vi "Receive Control Drop Event.vi"(8 "error in (no error)":errorcluster, 10 "ControlDropMsg":refnum<class "ControlDropMsg.lvclass">, 11 "IEventAggregator In":refnum<class "IEventAggregator.lvclass">) -> (0 "error out":errorcluster, 3 "IEventAggregator Out":refnum<class "IEventAggregator.lvclass">)   [LabVIEW 2020, in "ActorEvents.lvlib" / "IEventAggregator.lvclass"]
doc: "抽象方法\n接收控件放置事件"
uses:
  IEventAggregator.lvclass
  IEventAggregator Messages/ControlDropMsg/ControlDropMsg.lvclass
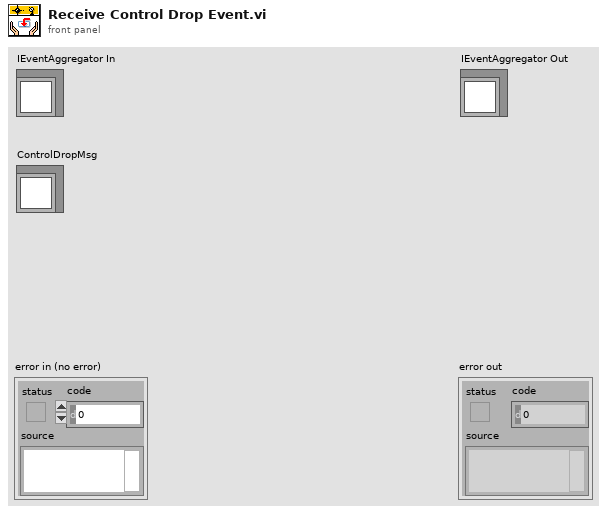
[diagram p1: front panel]
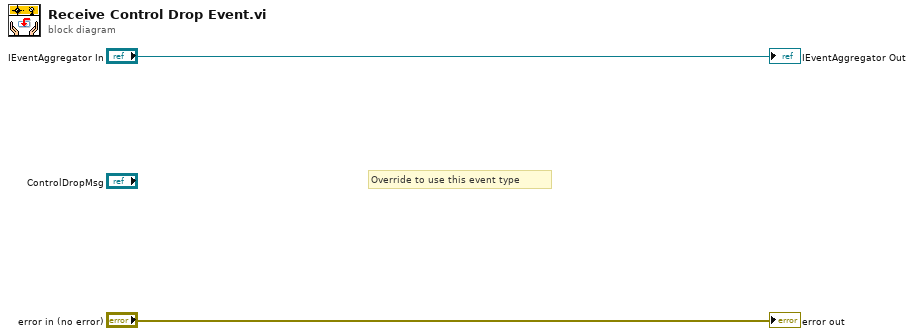
[diagram p0: block diagram]
diagram:
  # "Override to use this event type"
  "error out" <- "error in (no error)"
  "IEventAggregator Out" <- "IEventAggregator In"
